vi "Map.vi"(0 "Input":dbl, 2 "Input range":cluster{"Min":dbl, "Max":dbl}, 4 "Output range":cluster{"Min":dbl, "Max":dbl}) -> (5 "Output":dbl)   [LabVIEW 2014]
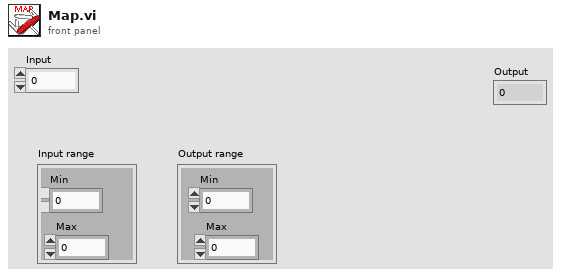
[diagram p1: front panel]
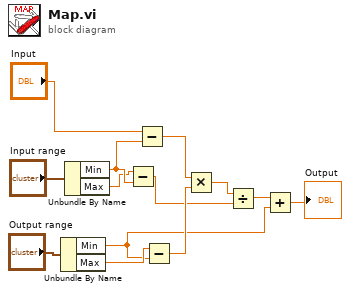
[diagram p0: block diagram]
diagram:
  n1 = Unbundle By Name("Output range") -> ("Min"=w1:dbl, "Max"=w2:dbl)
  n2 = Unbundle By Name("Input range") -> ("Min"=w4:dbl, "Max"=w3:dbl)
  n3 = Subtract(x=w3, y=w4) -> (x-y=w7:dbl)
  n4 = Subtract(x="Input", y=w4) -> (x-y=w10:dbl)
  n5 = Subtract(x=w2, y=w1) -> (x-y=w9:dbl)
  n6 = Multiply(x=w10, y=w9) -> (x*y=w8:dbl)
  n7 = Divide(x=w8, y=w7) -> (x/y=w6:dbl)
  n8 = Add(x=w6, y=w1) -> (x+y=→"Output":dbl)
